vi "templates ANALYSIS data keys.vi"(9 "Template Keys":T1, 10 "HTM Keys":T1) -> (2 "HTM Keys":T1)   [LabVIEW 2011]
uses:
  Addons/internet/utils/keyedarr.llb/Keyed Array.ctl
  Addons/internet/utils/strutil.llb/Case Matching.ctl
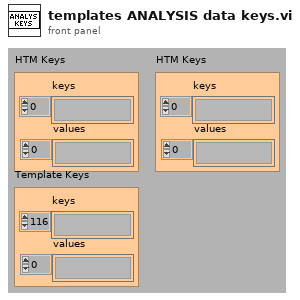
[diagram p1: front panel]
types:
  T1 = typedef "Keyed Array.ctl" = cluster{"keys":string[], "values":string[]}
  T2 = typedef "Case Matching.ctl" = enum16{"a != A", "a == A", "system"}
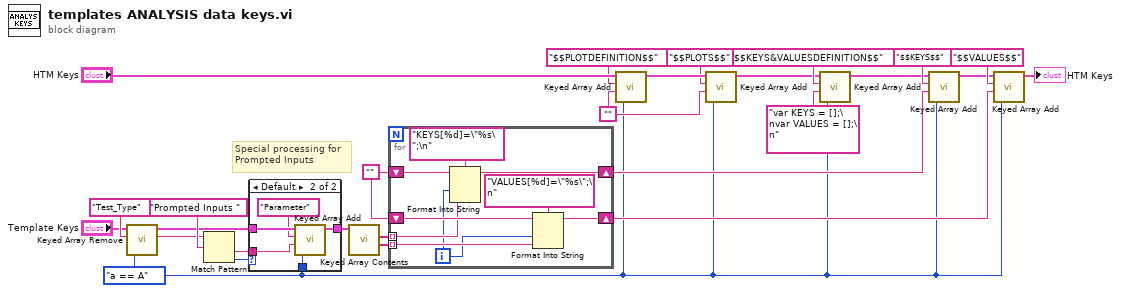
[diagram p0: block diagram]
diagram:
  w8 = ""
  w12 = ""
  w2 = Case_Matching."a == A" ("case matching (sensitive)")
  # "Special processing for\nPrompted Inputs"
  n1 = call "Keyed Array Remove.vi"("case matching (sensitive)"=w2, "key"="Test_Type" ("format string"), "array in"="Template Keys") -> ("value"=w6:string, "array out"=w5:T1)  [unwired: 3 out]
  n2 = Match Pattern(string=w6, regular expression="Prompted Inputs ") -> (after substring=w1:string, offset past match=w4:i32)  [unwired: 3 out]
  n3 = case shown="Default" w4 {
    tunnel: w5 -> [w28 w33]
    tunnel: [w28 w32] -> w3
    tunnel: w2 -> [_ w31]
    tunnel: w1 -> [_ w29]
    frame -1 {
    }
    frame Default {
      n4 = call "Keyed Array Add.vi"("case matching (sensitive)"=w31, "value"=w29, "key"="Parameter" ("regular expression"), "array in"=w33) -> ("array out"=w32:T1)  [unwired: 3 out]
    }
  }
  n5 = call "Keyed Array Contents.vi"("array in"=w3) -> ("values"=w13:string[], "keys"=w14:string[])  [unwired: 5 out]
  n6 = for {
    tunnel: w14 -> [w35] mode=indexing
    shift-right: [w41] -> w16
    shift-left: w8 -> [w42]
    tunnel: w13 -> [w40] mode=indexing
    shift-right: [w38] -> w15
    shift-left: w8 -> [w39]
    i -> [w34]
    n7 = Format Into String(format string="KEYS[%d]=\"%s\";\n", initial string=w42, w34, w35) -> (resulting string=w41:string)  [unwired: 1 in, 1 out]
    n8 = Format Into String(format string="VALUES[%d]=\"%s\";\n", initial string=w39, w34, w40) -> (resulting string=w38:string)  [unwired: 1 in, 1 out]
  }
  n9 = call "Keyed Array Add.vi"("case matching (sensitive)"=w2, "value"=w12, "key"="$$PLOTDEFINITION$$", "array in"="HTM Keys") -> ("array out"=w25:T1)  [unwired: 3 out]
  n10 = call "Keyed Array Add.vi"("case matching (sensitive)"=w2, "value"=w12, "key"="$$PLOTS$$", "array in"=w25) -> ("array out"=w17:T1)  [unwired: 3 out]
  n11 = call "Keyed Array Add.vi"("case matching (sensitive)"=w2, "value"="var KEYS = [];\nvar VALUES = [];\n" ("format string"), "key"="$$KEYS&VALUESDEFINITION$$", "array in"=w17) -> ("array out"=w20:T1)  [unwired: 3 out]
  n12 = call "Keyed Array Add.vi"("case matching (sensitive)"=w2, "value"=w16, "key"="$$KEYS$$", "array in"=w20) -> ("array out"=w19:T1)  [unwired: 3 out]
  n13 = call "Keyed Array Add.vi"("case matching (sensitive)"=w2, "value"=w15, "key"="$$VALUES$$", "array in"=w19) -> ("array out"=→"HTM Keys":T1)  [unwired: 3 out]
